vi "Handle Command.vi"(8 "error in (no error)":errorcluster, 10 "CMD in":refnum<class "Change Denuded Bypass State.lvclass">, 11 "Object In":refnum<class>) -> (0 "error out":errorcluster, 1 "Command Successful?":bool, 2 "CMD out":refnum<class "Change Denuded Bypass State.lvclass">, 3 "Object Out":refnum<class>)   [LabVIEW 2015, in "ePAS Library.lvlib" / "Change Denuded Bypass State.lvclass"]
doc: "This VI will contain the code used to actually execute the request. If the request is successful, this will be indicated by the boolean output <b>Command Successful?</b>. The boolean output can then be used by the <b>Command Reply</b> which sends a reply if the reply queue is valid."
uses:
  Change Denuded Bypass State.lvclass
  Instrument/ePAS.lvclass
  <vilib>/DAQmx/write.llb/DAQmx Write (Digital 1D Bool 1Chan 1Samp).vi
  reusable/Session APIs/Session Log/System Log.lvclass
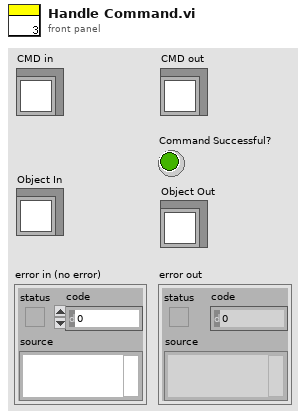
[diagram p1: front panel]
types:
  T1 = typedef "Session - Root.lvclass/Session Handle.ctl" = refnum<data-value>
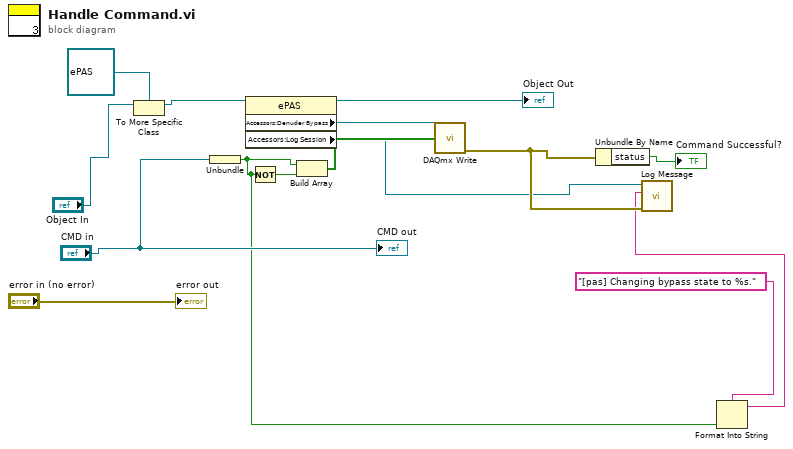
[diagram p0: block diagram]
diagram:
  n1 = To More Specific Class(target class=refnum<class "ePAS.lvclass"> refnum ("ePAS"), reference="Object In") -> (specific class reference=w12:refnum<class "ePAS.lvclass">)  [unwired: 1 in, 1 out]
  n2 = Unbundle("CMD in") -> (w4:bool)
  n3 = property class="ePAS"(reference=w12) -> (reference out=→"Object Out":refnum<class "ePAS.lvclass">, "Accessors:Denuder Bypass"=w10:refnum<k21>, "Accessors:Log Session"=w1:T1)  [unwired: 1 in, 1 out]
  n4 = Not(x=w4) -> (.not. x?=w8:bool)
  n5 = Build Array(w4, w8) -> (w7:bool[])
  n6 = call-poly <vilib>:"DAQmx Write.vi"("task/channels in"=w10, "data"=w7) -> ("error out"=w6:errorcluster)  [unwired: 11 in, 2 out]
  n7 = Unbundle By Name(w6) -> ("status"=→"Command Successful?":bool)
  n8 = Format Into String(format string="[pas] Changing bypass state to %s.", w4) -> (resulting string=w3:string)  [unwired: 2 in, 1 out]
  n9 = call "Log Message.vi"("error in"=w6, "MSG In"=w3, "session in"=w1) -> ()  [unwired: 7 in, 2 out]
  "error out" <- "error in (no error)"
  "CMD out" <- "CMD in"
